vi "Get Graph Properties.vi"(0 "WFGraph Refnum":refnum<vi>, 11 "error in (no error)":errorcluster) -> (4 "WFGraph Refnum (thru)":refnum<vi>, 8 "Graph Properties":T1, 15 "error out":errorcluster)   [LabVIEW 2020]
uses:
  Graph Properties.ctl
  Axis Properties.ctl
  Plot Properties.ctl
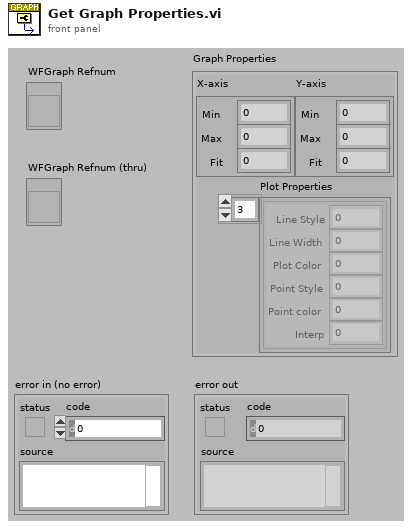
[diagram p1: front panel]
types:
  T1 = typedef "Graph Properties.ctl" = cluster{"X-axis":T2, "Y-axis":T2, "Plot Properties":T3[]}
  T2 = typedef "Axis Properties.ctl" = cluster{"Min":dbl, "Max":dbl, "Fit":u8}
  T3 = typedef "Plot Properties.ctl" = cluster{"Line Style":u8, "Line Width":u8, "Plot Color":u32, "Point Style":u8, "Point color":u32, "Interp":u8}
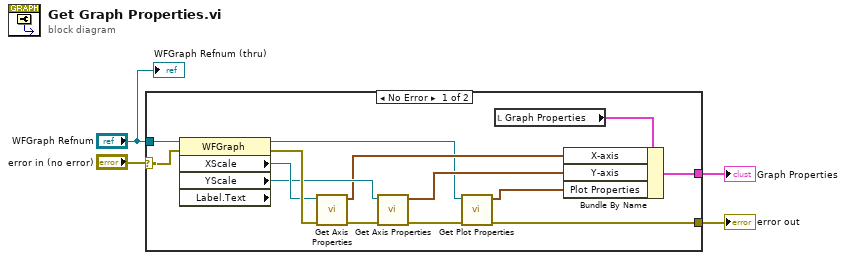
[diagram p0: block diagram]
diagram:
  n1 = case shown="No Error" "error in (no error)" {
    selector: "error in (no error)" -> [w17 w19]
    tunnel: "WFGraph Refnum" -> [w18 _]
    tunnel: [w6 w19] -> w3
    tunnel: [w5 _] -> w2
    frame No Error {
      n2 = property class="WFGraph" props=["XScale", "YScale", "Label", "Text"](reference=w18, error in=w17) -> (reference out=w9:refnum<vi>, error out=w16:errorcluster, "XScale"=w15:refnum<vi>, "YScale"=w13:refnum<vi>)  [unwired: 1 out]
      n3 = call "Get Axis Properties.vi"("error in (no error)"=w16, "Scale Refnum"=w15) -> ("error out"=w14:errorcluster, "Axis Properties"=w11:T2)  [unwired: 8 in]
      n4 = call "Get Axis Properties.vi"("error in (no error)"=w14, "Scale Refnum"=w13) -> ("error out"=w10:errorcluster, "Axis Properties"=w12:T2)  [unwired: 8 in]
      n5 = call "Get Plot Properties.vi"("error in (no error)"=w10, "Scale Refnum"=w9) -> ("error out"=w6:errorcluster, "Array"=w8:T3[])  [unwired: 8 in]
      n6 = local read "Graph Properties"() -> (w7:T1)
      n7 = Bundle By Name(cluster=w7, "X-axis"=w11, "Y-axis"=w12, "Plot Properties"=w8) -> (w5:T1)
    }
    frame Error {
    }
  }
  "error out" <- w3
  "Graph Properties" <- w2
  "WFGraph Refnum (thru)" <- "WFGraph Refnum"
